vi "PH_Beckhoff_StepMot.declare Sonderklemmen InputTags.vi"(2 "# of StepMot-Klemmen":i32=2, 3 "Instance Name":string="N/A") -> (0 "Sonderklemmen Inputs":T1, 1 "Description":string)   [LabVIEW 2014, in "PH_Beckhoff_StepMot.lvlib"]
uses:
  PH_Beckhoff_StepMot.lvlib
  PH_Beckhoff/PH_Beckhoff.Sonderklemmen Inputs.ctl
  PH_Beckhoff/PH_Beckhoff.lvlib
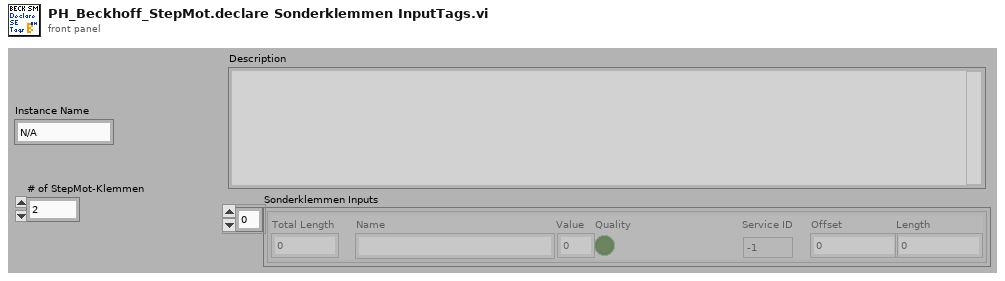
[diagram p1: front panel]
types:
  T1 = typedef "PH_Beckhoff.lvlib/PH_Beckhoff.Sonderklemmen Inputs.ctl" = cluster{"Total Length":u32, "Name":string, "Value":u64, "Quality":bool, "Service ID":i32, "Offset":u32, "Length":u32}[]
  T2 = cluster{"Total Length":u32, "Name":string, "Value":u32, "Quality":bool, "Service ID":i32, "Offset":u32, "Length":u32}
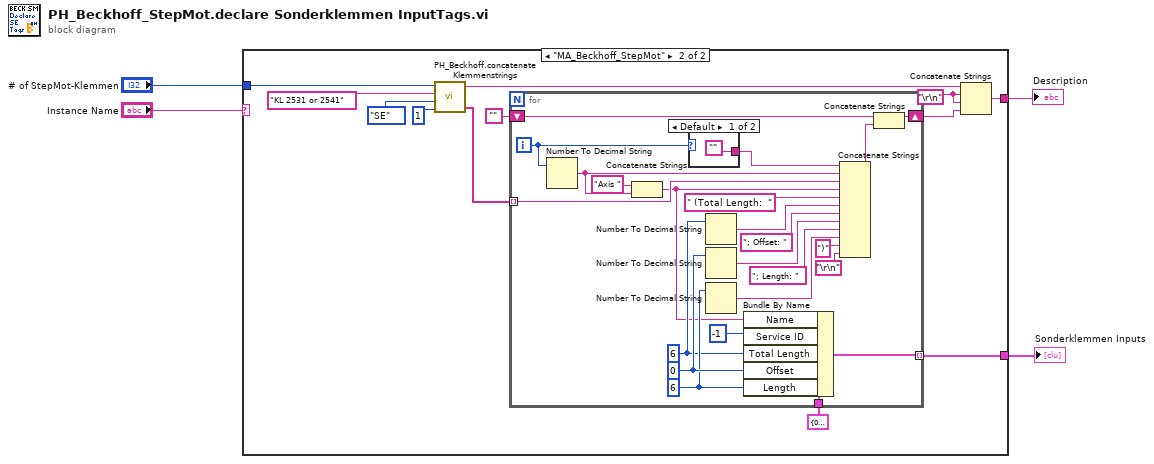
[diagram p0: block diagram]
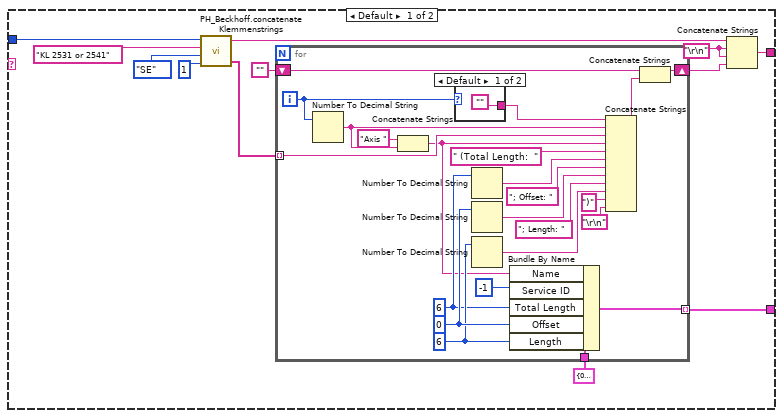
[diagram p2: hidden frame]
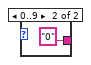
[diagram p3: hidden frame]
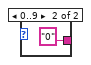
[diagram p4: hidden frame]
diagram:
  n1 = case shown="\"MA_Beckhoff_StepMot\"" "Instance Name" {
    tunnel: [w13 w50] -> w4
    tunnel: "# of StepMot-Klemmen" -> [w10 w47]
    tunnel: [w6 w43] -> w2
    frame Default {
      w14 = "\r\n"
      n2 = call "PH_Beckhoff.concatenate Klemmenstrings.vi"("# of In- or Outputs"=1, "Type"=enum16{"AE", "AA", "DE", "DA", "SE"}."SE", "Klemmenname"="KL 2531 or 2541", "Quantity"=w10) -> ("concatenated string array"=w8:string[], "\"<Type>: <Quantity> x <Klemmenname>\""=w9:string)  [unwired: 1 out]
      n3 = for {
        tunnel: w8 -> [w21] mode=indexing
        shift-right: [w36] -> w15
        shift-left: "" -> [w35]
        tunnel: T2 {"Total Length"=0, "Name"="", "Value"=0, "Quality"=FALSE, "Service ID"=0, "Offset"=0, "Length"=0} ("Input Value") -> [w33]
        tunnel: [w32] -> w6 mode=indexing
        i -> [w20]
        w25 = u32 6 ("Length")
        w22 = u32 6 ("Length")
        w31 = u32 0 ("Offset")
        n4 = Number To Decimal String(number=w20) -> (decimal integer string=w17:string)  [unwired: 1 in]
        n5 = Concatenate Strings("Axis " ("string"), w17) -> (w18:string)
        n6 = case shown="Default" w20 {
          tunnel: ["" "0"] -> w39
          frame Default {
          }
          frame 0..9 {
          }
        }
        n7 = Number To Decimal String(number=w22) -> (decimal integer string=w23:string)  [unwired: 1 in]
        n8 = Number To Decimal String(number=w31) -> (decimal integer string=w28:string)  [unwired: 1 in]
        n9 = Number To Decimal String(number=w25) -> (decimal integer string=w26:string)  [unwired: 1 in]
        n10 = Bundle By Name(cluster=w33, "Name"=w18, "Service ID"=-1, "Total Length"=w22, "Offset"=w31, "Length"=w25) -> (w32:T2)
        n11 = Concatenate Strings(w39, w17, w21, w18, " (Total Length:  " ("string"), w23, "; Offset: " ("string"), w28, "; Length: " ("string"), w26, ")" ("string"), "\r\n") -> (w37:string)
        n12 = Concatenate Strings(w35, w37) -> (w36:string)
      }
      n13 = Concatenate Strings(w9, w14, w14, w15) -> (w13:string)
    }
    frame "MA_Beckhoff_StepMot" {
      w51 = "\r\n"
      n14 = call "PH_Beckhoff.concatenate Klemmenstrings.vi"("# of In- or Outputs"=1, "Type"=enum16{"AE", "AA", "DE", "DA", "SE"}."SE", "Klemmenname"="KL 2531 or 2541", "Quantity"=w47) -> ("concatenated string array"=w45:string[], "\"<Type>: <Quantity> x <Klemmenname>\""=w46:string)  [unwired: 1 out]
      n15 = for {
        tunnel: w45 -> [w58] mode=indexing
        shift-right: [w73] -> w52
        shift-left: "" -> [w72]
        tunnel: T2 {"Total Length"=0, "Name"="", "Value"=0, "Quality"=FALSE, "Service ID"=0, "Offset"=0, "Length"=0} ("Input Value") -> [w70]
        tunnel: [w69] -> w43 mode=indexing
        i -> [w57]
        w62 = u32 6 ("Length")
        w59 = u32 6 ("Length")
        w68 = u32 0 ("Offset")
        n16 = Number To Decimal String(number=w57) -> (decimal integer string=w54:string)  [unwired: 1 in]
        n17 = Concatenate Strings("Axis " ("string"), w54) -> (w55:string)
        n18 = case shown="Default" w57 {
          tunnel: ["" "0"] -> w76
          frame Default {
          }
          frame 0..9 {
          }
        }
        n19 = Number To Decimal String(number=w59) -> (decimal integer string=w60:string)  [unwired: 1 in]
        n20 = Number To Decimal String(number=w68) -> (decimal integer string=w65:string)  [unwired: 1 in]
        n21 = Number To Decimal String(number=w62) -> (decimal integer string=w63:string)  [unwired: 1 in]
        n22 = Bundle By Name(cluster=w70, "Name"=w55, "Service ID"=-1, "Total Length"=w59, "Offset"=w68, "Length"=w62) -> (w69:T2)
        n23 = Concatenate Strings(w76, w54, w58, w55, " (Total Length:  " ("string"), w60, "; Offset: " ("string"), w65, "; Length: " ("string"), w63, ")" ("string"), "\r\n") -> (w74:string)
        n24 = Concatenate Strings(w72, w74) -> (w73:string)
      }
      n25 = Concatenate Strings(w46, w51, w51, w52) -> (w50:string)
    }
  }
  "Description" <- w4
  "Sonderklemmen Inputs" <- w2
